vi "Process.vi"(8 "error in (no error)":errorcluster, 10 "Pound in":refnum<class "Pound.lvclass">, 11 "Qbus in":refnum<class "Qbus.lvclass">) -> (0 "error out":errorcluster)   [LabVIEW 2017, in "CmsFpgaBitfileManager.lvlib"]
doc: "This process downloads the appropriate bitfile to the device FPGA so it can begin to acquire data. For example, the Scan Engine process cannot begin to acquire data until the FPGA bitfile is downloaded."
uses:
  <vilib>/addons/InsightCM/Devices/Shared/Cms/CmsFpgaBitfileManager/CmsFpgaBitfileManager.lvlib
  <vilib>/addons/Qbus/Qbus.lvclass
  <vilib>/NI/Software Watchdog/Pound/Pound.lvclass
  <vilib>/addons/InsightCM/Devices/Shared/Cms/CmsFpgaBitfileManager/controls/config.ctl
  <vilib>/FPGAPlugInAG/Dynamic/niLvFpga_Close_Dynamic.vi
  <vilib>/rvi/interface/nirviCloseFPGA/nirviCloseFPGA.xnode
  <vilib>/addons/TraceLogger/TraceLogger.lvlib
  <vilib>/NI/Software Watchdog/Watchdog/Watchdog.lvclass
  <vilib>/addons/InsightCM/Devices/Shared/Common/FpgaBitfileManager/FpgaBitfileManager.lvlib
  <vilib>/addons/InsightCM/Utilities/GlobalConfiguration/GlobalConfiguration.lvlib
  <vilib>/addons/TimerProcess/TimerProcess.lvlib
  <vilib>/addons/TimerProcess/controls/taskType.ctl
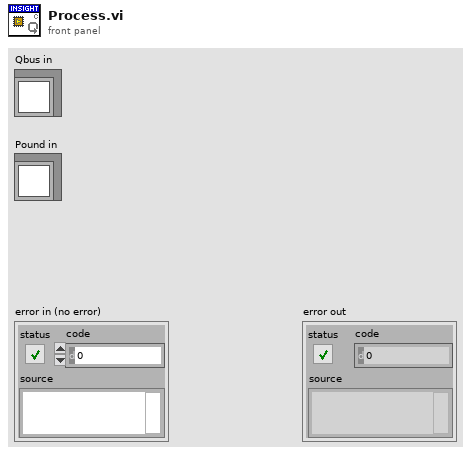
[diagram p1: front panel]
types:
  T1 = typedef "CmsFpgaBitfileManager.lvlib/config.ctl" = cluster{"Bitfile reference":refnum<k20>}
  T2 = typedef "TimerProcess.lvlib/taskType.ctl" = enum16{"single", "repeat"}
  T3 = typedef "cRIODetectHW.lvlib/SystemHW.ctl" = cluster{"controller":T4, "chassis":T4, "modules":T4[]}
  T4 = typedef "cRIODetectHW.lvlib/cRIO Product Info.ctl" = cluster{"vendorName":string, "productName":string, "serialNumber":string}
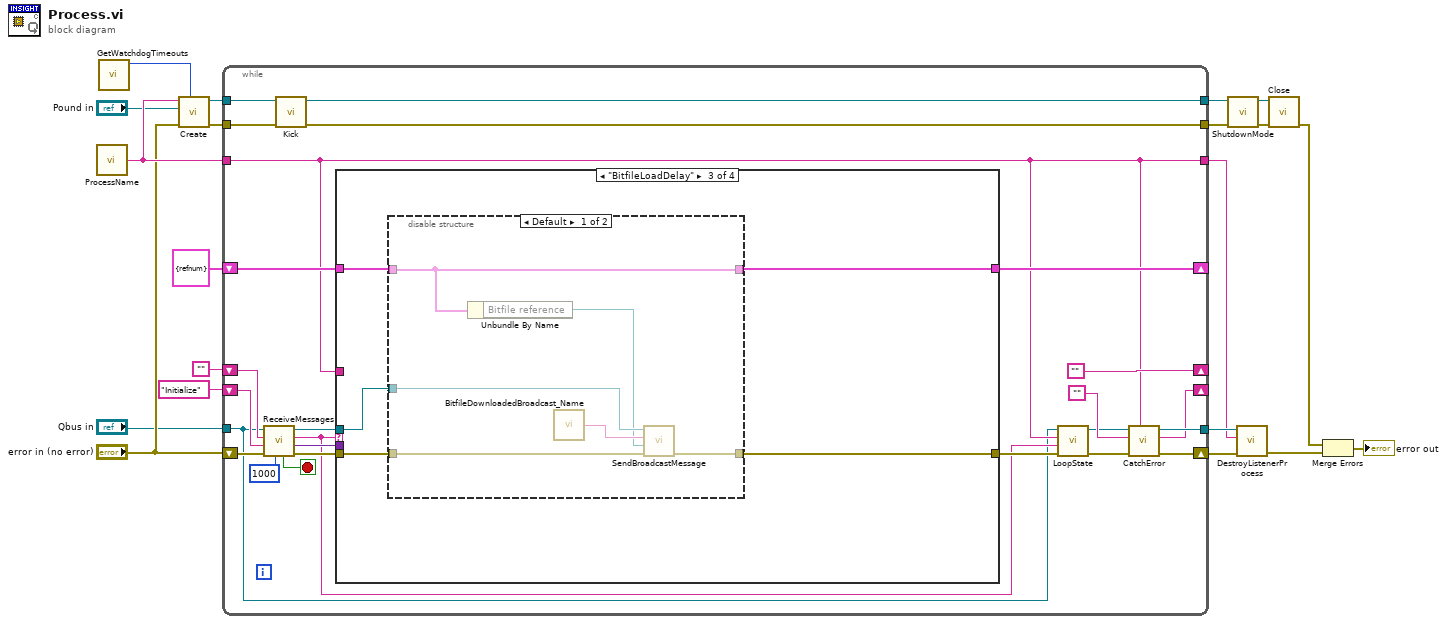
[diagram p0: block diagram]
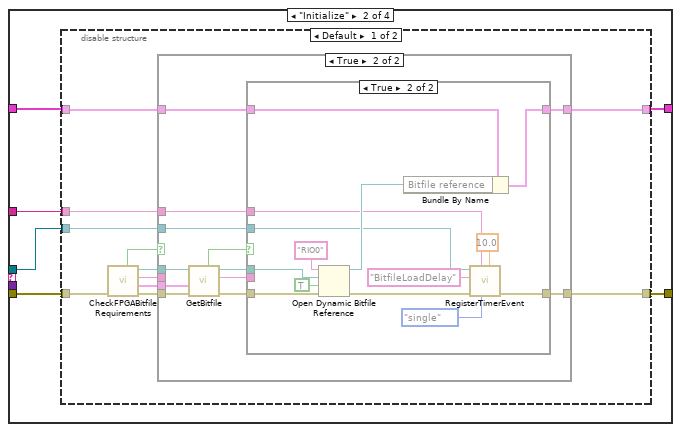
[diagram p3: hidden frame]
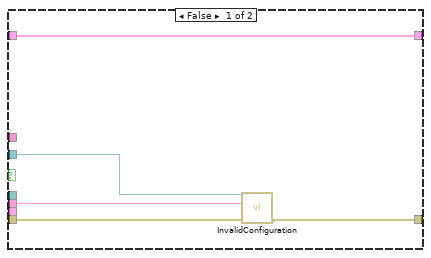
[diagram p4: hidden frame]
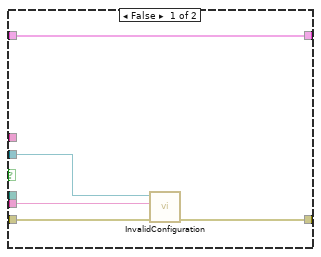
[diagram p5: hidden frame]
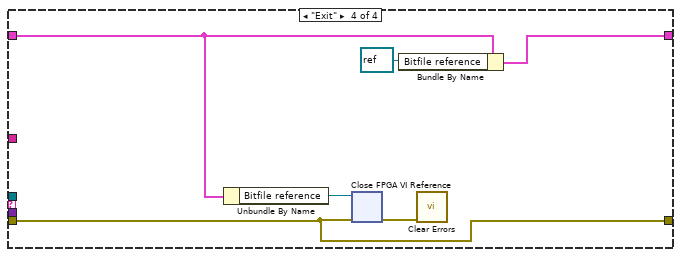
[diagram p8: hidden frame]
diagram:
  n1 = call <vilib>:"ProcessName.vi"() -> ("process name"=w14:string)  [unwired: 5 in]
  n2 = call <vilib>:"GetWatchdogTimeouts.vi"() -> ("software timeout"=w1:u32)  [unwired: 10 in, 1 out]
  n3 = call <vilib>:"Create.vi"("Execution Timeout (ms)"=w1, "error in (no error)"="error in (no error)", "Pound"="Pound in", "Name"=w14) -> ("error out"=w8:errorcluster, "Watchdog"=w13:refnum<data-value>)  [unwired: 6 in]
  n4 = while {
    shift-right: [""] -> _
    shift-left: "" -> [w44]
    tunnel: "Qbus in" -> [w24]
    tunnel: w14 -> [w31]
    tunnel: [w35] -> w18
    tunnel: [w31] -> w17
    shift-right: [w33] -> _
    shift-left: "Initialize" -> [w39]
    shift-right: [w37] -> _
    shift-left: T1 {"Bitfile reference"=refnum} ("config") -> [w38]
    tunnel: w13 -> [w30]
    tunnel: [w29] -> w10
    tunnel: w8 -> [w28]
    tunnel: [w26] -> w7
    shift-right: [w36] -> w19
    shift-left: "error in (no error)" -> [w27]
    stop <- w45 stop-if-true
    n5 = call <vilib>:"ReceiveMessages.vi"("timeout(1000)"=1000 ("Timeout(100)"), "error in (no error)"=w27, "priority action"=w39, "default action"=w44, "Qbus in"=w24) -> ("error out"=w43:errorcluster, "message value"=w40:variant, "action"=w25:string, "Qbus out"=w41:refnum<class "Qbus.lvclass">, "exit"=w45:bool)  [unwired: 2 in]
    n6 = call <vilib>:"Kick.vi"("error in (no error)"=w28, "Watchdog"=w30) -> ("error out"=w26:errorcluster, "Watchdog"=w29:refnum<data-value>)  [unwired: 8 in]
    n7 = case shown="\"BitfileLoadDelay\"" w25 {
      tunnel: w43 -> [w47 w49 w103 w119]
      tunnel: w41 -> [_ w50 w104 _]
      tunnel: [w47 w51 w105 w119] -> w32
      tunnel: w40 -> [_ _ _ _]
      tunnel: w38 -> [w46 w53 w107 w121]
      tunnel: [w46 w52 w106 w120] -> w37
      tunnel: w31 -> [_ w48 _ _]
      frame "", Default {
      }
      frame "Initialize" {
        n8 = disable-structure shown="Default" {
          disable-tunnel: w49 -> [w60 w101]
          disable-tunnel: w53 -> [w64 w102]
          disable-tunnel: [w63 w102] -> w52
          disable-tunnel: [w62 w101] -> w51
          disable-tunnel: w50 -> [w61 _]
          disable-tunnel: w48 -> [w54 _]
          frame condition #0 {
            n9 = call <vilib>:"CheckFPGABitfileRequirements.vi"("error in (no error)"=w60) -> ("error out"=w59:errorcluster, "system info"=w55:T3, "description"=w56:string, "bitfile dir"=w57:path, "valid"=w58:bool)  [unwired: 6 in]
            n10 = case shown="True" w58 {
              tunnel: w57 -> [_ w75]
              tunnel: w59 -> [w68 w79]
              tunnel: [w67 w81] -> w62
              tunnel: w64 -> [w69 w74]
              tunnel: [w69 w73] -> w63
              tunnel: w61 -> [w66 w80]
              tunnel: w56 -> [w65 _]
              tunnel: w55 -> [_ w77]
              tunnel: w54 -> [_ w70]
              frame False {
                n11 = call <vilib>:"InvalidConfiguration.vi"("error in (no error)"=w68, "description"=w65, "Qbus in"=w66) -> ("error out"=w67:errorcluster)  [unwired: 7 in, 1 out]
              }
              frame True {
                n12 = call <vilib>:"GetBitfile.vi"("error in (no error)"=w79, "system info"=w77, "bitfile dir"=w75) -> ("error out"=w78:errorcluster, "source"=w76:string, "Bitfile"=w71:path, "found"=w72:bool)  [unwired: 5 in]
                n13 = case shown="True" w72 {
                  tunnel: [w84 w92] -> w81
                  tunnel: w80 -> [w86 w91]
                  tunnel: w78 -> [w85 w98]
                  tunnel: w76 -> [w82 _]
                  tunnel: w74 -> [w83 w97]
                  tunnel: [w83 w96] -> w73
                  tunnel: w71 -> [_ w95]
                  tunnel: w70 -> [_ w90]
                  frame False {
                    n14 = call <vilib>:"InvalidConfiguration.vi"("error in (no error)"=w85, "description"=w82, "Qbus in"=w86) -> ("error out"=w84:errorcluster)  [unwired: 7 in, 1 out]
                  }
                  frame True {
                    n15 = Open Dynamic Bitfile Reference(0:"RIO0" ("Device address"), 1:w95, 2:TRUE ("Run When Loaded"), 3:w98) -> (5:w94:refnum<k20>, 8:w93:errorcluster)  [unwired: 1 in]
                    n16 = Bundle By Name(cluster=w97, "Bitfile reference"=w94) -> (w96:T1)
                    n17 = call <vilib>:"RegisterTimerEvent.vi"("interval (sec)"=10.0, "type"=taskType."single", "process name"=w90, "error in (no error)"=w93, "callback action"="BitfileLoadDelay", "qbus in"=w91) -> ("error out"=w92:errorcluster)  [unwired: 4 in, 1 out]
                  }
                }
              }
            }
          }
          frame condition #1 (active) {
          }
        }
      }
      frame "BitfileLoadDelay" {
        n18 = disable-structure shown="Default" {
          disable-tunnel: w103 -> [w108 w114]
          disable-tunnel: w107 -> [w109 w115]
          disable-tunnel: [w109 w115] -> w106
          disable-tunnel: [w113 w114] -> w105
          disable-tunnel: w104 -> [w112 _]
          frame condition #0 {
            n19 = Unbundle By Name(w109) -> ("Bitfile reference"=w110:refnum<k20>)
            n20 = call <vilib>:"BitfileDownloadedBroadcast_Name.vi"() -> ("message name"=w111:string)  [unwired: 5 in]
            n21 = call <vilib>:"SendBroadcastMessage.vi"("error in (no error)"=w108, "message value"=w110, "message name"=w111, "Qbus in"=w112) -> ("error in (no error)"=w113:errorcluster)  [unwired: 6 in, 1 out]
          }
          frame condition #1 (active) {
          }
        }
      }
      frame "Exit" {
        n22 = Unbundle By Name(w121) -> ("Bitfile reference"=w118:refnum<k20>)
        n23 = xnode "Close FPGA VI Reference"("FPGA VI Reference In"=w118, "error in"=w119) -> ("error out"=w116:errorcluster)
        n24 = Bundle By Name(cluster=w121, "Bitfile reference"=refnum<k20> refnum) -> (w120:T1)
        n25 = call <vilib>:"Clear Errors.vi"("error in (no error)"=w116) -> ()  [unwired: 5 in, 2 out]
      }
    }
    n26 = call <vilib>:"LoopState.vi"("error in (no error)"=w32, "loop action"=w25, "process name"=w31, "Qbus in"=w24) -> ("error out"=w22:errorcluster, "Qbus out"=w21:refnum<class "Qbus.lvclass">)  [unwired: 6 in]
    n27 = call <vilib>:"CatchError.vi"("source"=w31, "error in (no error)"=w22, "next action in"="", "Qbus in"=w21) -> ("error out"=w36:errorcluster, "next action out"=w33:string, "Qbus out"=w35:refnum<class "Qbus.lvclass">)  [unwired: 5 in]
  }
  n28 = call <vilib>:"ShutdownMode.vi"("error in (no error)"=w7, "Watchdog"=w10) -> ("error out"=w9:errorcluster, "Watchdog"=w11:refnum<data-value>)  [unwired: 8 in]
  n29 = call <vilib>:"DestroyListenerProcess.vi"("error in (no error)"=w19, "process name"=w17, "Qbus in"=w18) -> ("error in (no error)"=w6:errorcluster)  [unwired: 7 in, 1 out]
  n30 = call <vilib>:"Close.vi"("error in (no error)"=w9, "Watchdog"=w11) -> ("error out"=w5:errorcluster)  [unwired: 9 in]
  n31 = Merge Errors(w5, w6) -> (→"error out":errorcluster)
